vi "teleopVars.vi"() -> ()   [LabVIEW 2016]
panel:
  out "gearStatus":bool
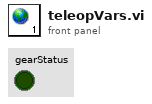
[diagram p1: front panel]
diagram:
